vi "Syslog Interface PC.vi"(8 "Fehler (in)":errorcluster caption="Fehlereingang", 11 "Cluster (in)":T1={"FehlermeldungsCode"=-1, "ErfolgsmeldungsCode"=-1, "ParameterListenString"="", "Anzeige"=FALSE, "SysLogIcon"=enum."OK", "intern"=FALSE}) -> (0 "Fehler (out)":errorcluster caption="Fehlerausgang")   [LabVIEW 2020, in "SysLog.lvlib"]
doc: "Interface zur Fehlerbehandlung PC\nFehler (Fehlereingang) wird in die #ErrorLogHistory aufgenommen.\nFehlermeldung wird übersetzt, wenn Sprach Index Seite oder Sprachliste angeschlossen sind.\nWenn Anzeige eingeschaltet, wird die Fehleranzeige aufgepoppt (nicht blockierend).\nErfolgsmeldung optional - wird dann ebenfalls geloggt, und wenn Anzeige eingeschaltet auch angezeigt.\nriw - 11.06.2018"
uses:
  SysLog.lvlib
  SysLog Interface.ctl
  Seiten/System Einstellungen V2/Aktioen FGV System Konstanten.ctl
  Aktionen FGV SysLog.ctl
  Allgemein/allgemeine Sub-VIs.lvlib
  Seiten/System Einstellungen V2/System Einstellungen V2.lvlib
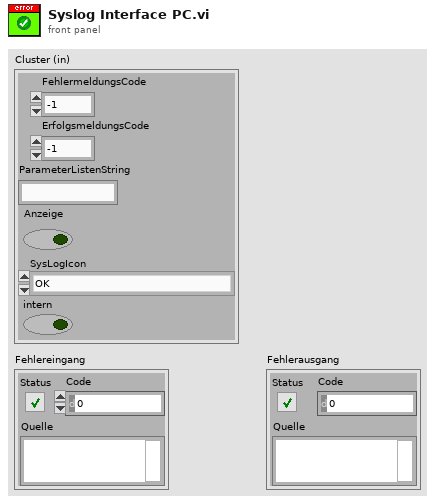
[diagram p1: front panel]
types:
  T1 = typedef "SysLog.lvlib/SysLog Interface.ctl" = cluster{"FehlermeldungsCode":i32, "ErfolgsmeldungsCode":i32, "ParameterListenString":string, "Anzeige":bool, "SysLogIcon":enum16{"OK", "Warnung", "Fehler"}, "intern":bool}
  T2 = typedef "System Einstellungen V2.lvlib/Aktioen FGV System Konstanten.ctl" = enum16{"lesen", "laden", "speichern", "Sprache"}
  T3 = typedef "SysLog.lvlib/Aktionen FGV SysLog.ctl" = enum16{"initialisieren", "lesen", "schreiben", "history button ref", "Syslog_Anforderung"}
  T4 = cluster{string, "Anzeige":bool, "SysLogIcon":enum16{"OK", "Warnung", "Fehler"}, "intern":bool}
  T5 = cluster{"Anzeige Array":bool[], "Message Array":string[], "SysLog Incon Array":enum16{"OK", "Warnung", "Fehler"}[], "Status Message Array":string[], "Status SysLog Incon Array":enum16{"OK", "Warnung", "Fehler"}[]}
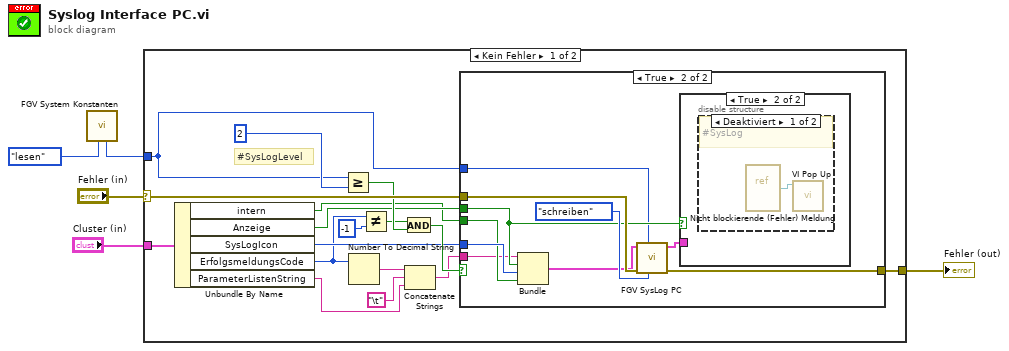
[diagram p0: block diagram]
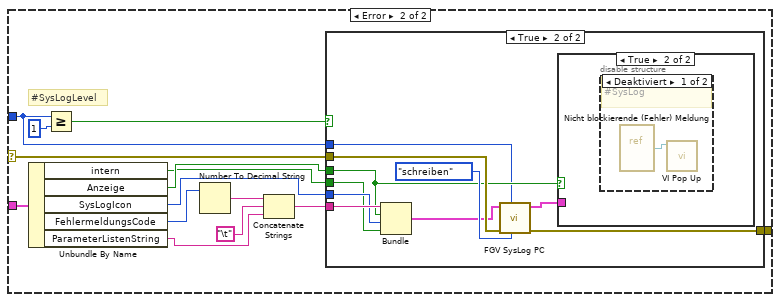
[diagram p5: hidden frame]
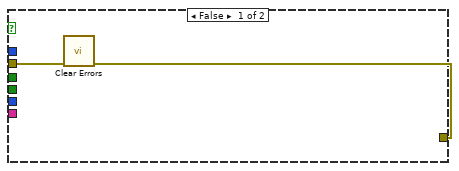
[diagram p6: hidden frame]
diagram:
  n1 = call "FGV System Konstanten.vi"("Aktionen"=Aktioen_FGV_System_Konstanten."lesen") -> ("SysLogLevel"=w2:u32)  [unwired: 6 in, 4 out]
  n2 = case shown="Kein Fehler" "Fehler (in)" {
    selector: "Fehler (in)" -> [w21 w47]
    tunnel: "Cluster (in)" -> [w22 w48]
    tunnel: w2 -> [w14 w42]
    tunnel: [w16 w46] -> w1
    frame No Error {
      # "#SysLogLevel"
      n3 = Unbundle By Name(w22) -> ("intern"=w12:bool, "Anzeige"=w13:bool, "SysLogIcon"=w15:enum16{"OK", "Warnung", "Fehler"}, "ErfolgsmeldungsCode"=w8:i32, "ParameterListenString"=w7:string)
      n4 = Greater Or Equal?(x=w14, y=u32 2) -> (x >= y?=w19:bool)
      n5 = Number To Decimal String(number=w8) -> (decimal integer string=w9:string)  [unwired: 1 in]
      n6 = Not Equal?(x=w8, y=-1) -> (x != y?=w18:bool)
      n7 = And(x=w18, y=w19) -> (x .and. y?=w17:bool)
      n8 = Concatenate Strings(w9, "\t", w7) -> (w6:string)
      n9 = case shown="True" w17 {
        tunnel: w21 -> [w23 w33]
        tunnel: w13 -> [_ w30]
        tunnel: [w23 w31] -> w16
        tunnel: w15 -> [_ w29]
        tunnel: w14 -> [_ w27]
        tunnel: w12 -> [_ w26]
        tunnel: w6 -> [_ w24]
        frame False {
        }
        frame True {
          n10 = Bundle(w24, "Anzeige"=w30, "SysLogIcon"=w29, "intern"=w26) -> (w28:T4)  [unwired: 1 in]
          n11 = call "FGV SysLog PC.vi"("Aktion"=Aktionen_FGV_SysLog."schreiben", "SysLogLevel"=w27, "Fehler (in)"=w33, "Cluster  (in)"=w28) -> ("Fehler (out)"=w31:errorcluster, "Anzeige Cluster"=w25:T5)  [unwired: 3 in, 3 out]
          n12 = case shown="True" w30 {
            tunnel: w25 -> [_ _]
            frame False {
            }
            frame True {
              n13 = disable-structure shown="Deaktiviert" {
                frame Disabled {
                  # "#SysLog"
                  n14 = vi-ref "Nicht blockierende (Fehler) Meldung.vi"() -> (w34:refnum<vi>)
                  n15 = call "VI Pop Up.vi"("VI Referenz"=w34) -> ()  [unwired: 11 in]
                }
                frame Enabled {
                }
              }
            }
          }
        }
      }
    }
    frame Error {
      # "#SysLogLevel"
      n16 = Unbundle By Name(w48) -> ("intern"=w40:bool, "Anzeige"=w41:bool, "SysLogIcon"=w43:enum16{"OK", "Warnung", "Fehler"}, "FehlermeldungsCode"=w37:i32, "ParameterListenString"=w36:string)
      n17 = Greater Or Equal?(x=w42, y=u32 1) -> (x >= y?=w44:bool)
      n18 = Number To Decimal String(number=w37) -> (decimal integer string=w39:string)  [unwired: 1 in]
      n19 = Concatenate Strings(w39, "\t", w36) -> (w35:string)
      n20 = case shown="True" w44 {
        tunnel: w35 -> [_ w60]
        tunnel: w47 -> [w50 w58]
        tunnel: w41 -> [_ w56]
        tunnel: [w49 w57] -> w46
        tunnel: w43 -> [_ w55]
        tunnel: w42 -> [_ w53]
        tunnel: w40 -> [_ w52]
        frame False {
          n21 = call <vilib>:"Clear Errors.vi"("error in (no error)"=w50) -> ("error out"=w49:errorcluster)  [unwired: 5 in, 1 out]
        }
        frame True {
          n22 = Bundle(w60, "Anzeige"=w56, "SysLogIcon"=w55, "intern"=w52) -> (w54:T4)  [unwired: 1 in]
          n23 = call "FGV SysLog PC.vi"("Aktion"=Aktionen_FGV_SysLog."schreiben", "SysLogLevel"=w53, "Fehler (in)"=w58, "Cluster  (in)"=w54) -> ("Fehler (out)"=w57:errorcluster, "Anzeige Cluster"=w51:T5)  [unwired: 3 in, 3 out]
          n24 = case shown="True" w56 {
            tunnel: w51 -> [_ _]
            frame False {
            }
            frame True {
              n25 = disable-structure shown="Deaktiviert" {
                frame Disabled {
                  # "#SysLog"
                  n26 = vi-ref "Nicht blockierende (Fehler) Meldung.vi"() -> (w61:refnum<vi>)
                  n27 = call "VI Pop Up.vi"("VI Referenz"=w61) -> ()  [unwired: 11 in]
                }
                frame Enabled {
                }
              }
            }
          }
        }
      }
    }
  }
  "Fehler (out)" <- w1
